vi "15_01_2021.vi"() -> ()   [LabVIEW 2020]
panel:
  out "Numeric 3":dbl
  in  "Valor 2":dbl
  in  "Boolean":bool
  in  "Valor 1":dbl
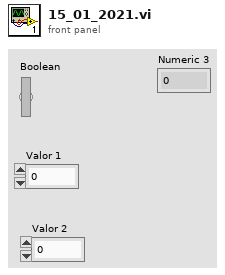
[diagram p1: front panel]
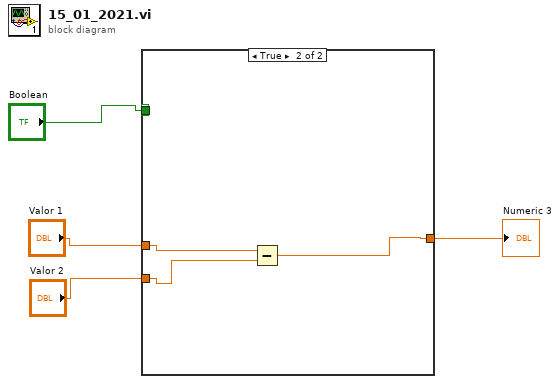
[diagram p0: block diagram]
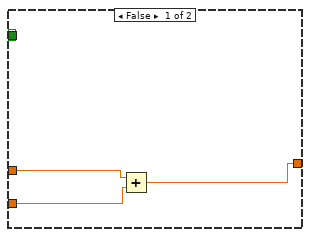
[diagram p2: hidden frame]
diagram:
  n1 = case shown="True" "Boolean" {
    selector: "Boolean" -> [w6 _]
    tunnel: "Valor 1" -> [w8 w11]
    tunnel: "Valor 2" -> [w7 w10]
    tunnel: [w6 _] -> _
    tunnel: [w5 w9] -> w1
    frame False {
      n2 = Add(x=w8, y=w7) -> (x+y=w5:dbl)
    }
    frame True {
      n3 = Subtract(x=w11, y=w10) -> (x-y=w9:dbl)
    }
  }
  "Numeric 3" <- w1
